vi "CSMOMgr-Delete.vi"(8 "Error in":errorcluster caption="Error in (no error)", 10 "Queue Name":string, 11 "CSMOMgr":T1) -> (0 "Error out":errorcluster, 3 "CSMOMgr out":T1)   [LabVIEW 2014, in "Communicable State Machine.lvlib"]
uses:
  Communicable State Machine.lvlib
  Def-CSMOMgr.ctl
  CSMQ/_CSMObj.ctl
  Typedef/_CSM_MODE.ctl
  Priority Queue/Priority Queue.lvclass
  CSMQ/_CSMObj-Data.ctl
  Typedef/_CSM Status Change Event Data.ctl
  FGV-BroadcastRegistry/Operation-BroadcastRegistry.ctl
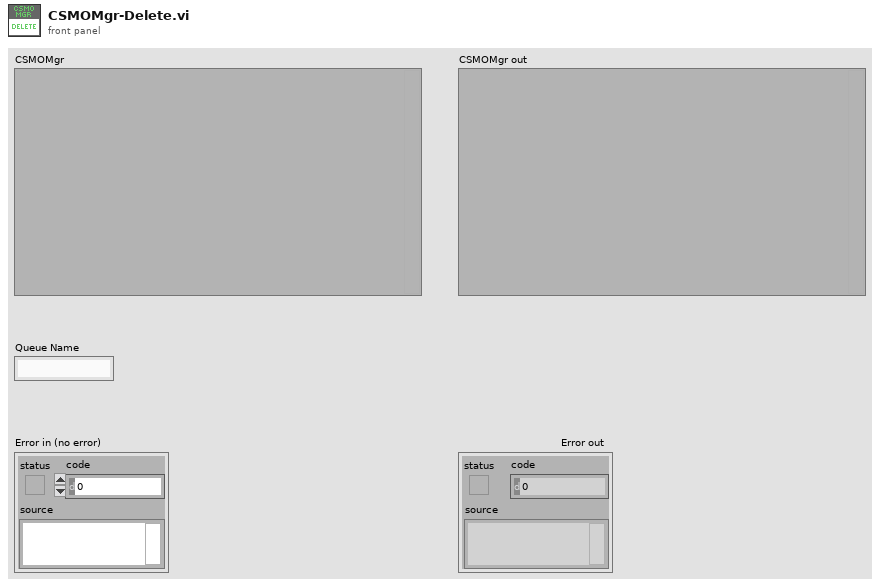
[diagram p1: front panel]
types:
  T1 = typedef "Communicable State Machine.lvlib/Def-CSMOMgr.ctl" = variant
  T2 = typedef "Communicable State Machine.lvlib/_CSMObj.ctl" = cluster{"Queue Name":string, "Mode":T3, "Share Count":i32, "Queue":refnum<class "Priority Queue.lvclass">, "Locked Status":refnum<data-value>, "User Event":refnum<user-event>, "Status Change Event":refnum<user-event>, "Allowed Messages":string[]}
  T3 = typedef "Communicable State Machine.lvlib/_CSM_MODE.ctl" = enum16{"Stand Alone", "CSM", "Action Worker", "Responsibility Chain", "Responsibility Chain Node"}
  T4 = typedef "Communicable State Machine.lvlib/Operation-BroadcastRegistry.ctl" = enum16{"Delete Source Module", "Delete Target Module", "Remove Module", "Register", "Unregister", "Check"}
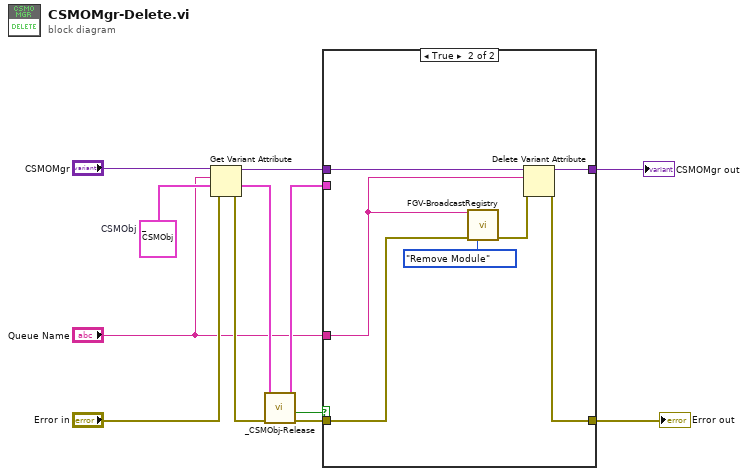
[diagram p0: block diagram]
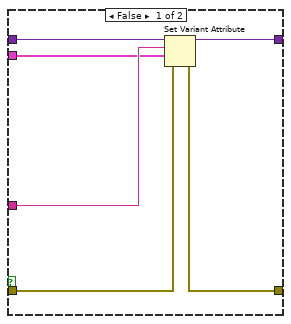
[diagram p2: hidden frame]
diagram:
  w2 = T2 {"Queue Name"="", "Mode"=enum."Stand Alone", "Share Count"=0, "Queue"=refnum, "Locked Status"=refnum, "User Event"=refnum, "Status Change Event"=refnum, "Allowed Messages"=[]}  # CSMObj
  n1 = Get Variant Attribute(Variant="CSMOMgr", name="Queue Name", default value (empty Variant)=w2, error in="Error in") -> (duplicate Variant=w12:variant, value=w11:T2, error out=w7:errorcluster)  [unwired: 1 out]
  n2 = call "_CSMObj-Release.vi"("Error in"=w7, "CSMQ in"=w11) -> ("Error out"=w8:errorcluster, "Release?"=w10:bool, "CSMQ out"=w9:T2)  [unwired: 7 in]
  n3 = case shown="True" w10 {
    tunnel: "Queue Name" -> [w16 w22]
    tunnel: w12 -> [w18 w24]
    tunnel: [w17 w23] -> w5
    tunnel: w9 -> [w15 _]
    tunnel: w8 -> [w14 w21]
    tunnel: [w13 w19] -> w3
    frame False {
      n4 = Set Variant Attribute(Variant=w18, name=w16, value=w15, error in=w14) -> (Variant out=w17:variant, error out=w13:errorcluster)  [unwired: 1 out]
    }
    frame True {
      n5 = call "FGV-BroadcastRegistry.vi"("Source"=w22, "Error in"=w21, "Operation"=Operation-BroadcastRegistry."Remove Module") -> ("Error out"=w20:errorcluster)  [unwired: 10 in, 2 out]
      n6 = Delete Variant Attribute(4:w20, 6:w22, 7:w24) -> (0:w19:errorcluster, 3:w23:variant)  [unwired: 1 out]
    }
  }
  "Error out" <- w3
  "CSMOMgr out" <- w5
